vi "Timed Messaging_Skip.vi"(9 "expected":i32=5, 10 "notification":T1=enum."Send next copy now and stop all further copies") -> (3 "Pass?":bool)   [LabVIEW 2014]
uses:
  <vilib>/ActorFramework/Message/Message.lvclass
  <vilib>/ActorFramework/Time-Delayed Send Message/Time-Delay Override Options.ctl
  Increment Msg/Increment Msg.lvclass/Increment Msg.ctl
  <vilib>/ActorFramework/Message Queue/Message Queue.lvclass/Message Queue.ctl
  <vilib>/ActorFramework/Message Dequeuer/Message Dequeuer.lvclass/Message Dequeuer.ctl
  <vilib>/ActorFramework/Message Priority Queue/Priority Dequeue.vi
  Increment Msg/Increment Msg.lvclass
  <vilib>/ActorFramework/Message Queue/Message Queue.lvclass
  <vilib>/ActorFramework/Message Dequeuer/Message Dequeuer.lvclass
panel:
  out "Array":refnum<class "Message.lvclass">[](array[class])
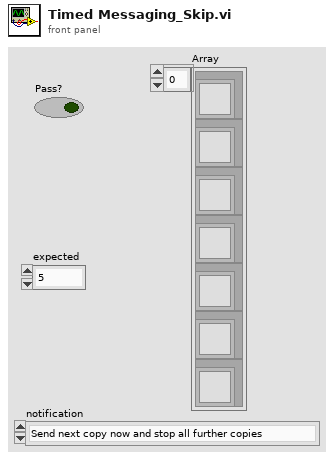
[diagram p1: front panel]
types:
  T1 = typedef "Time-Delay Override Options.ctl" = enum16{"Send next copy now", "Skip next scheduled copy", "Send next copy now and stop all further copies", "Stop all further copies"}
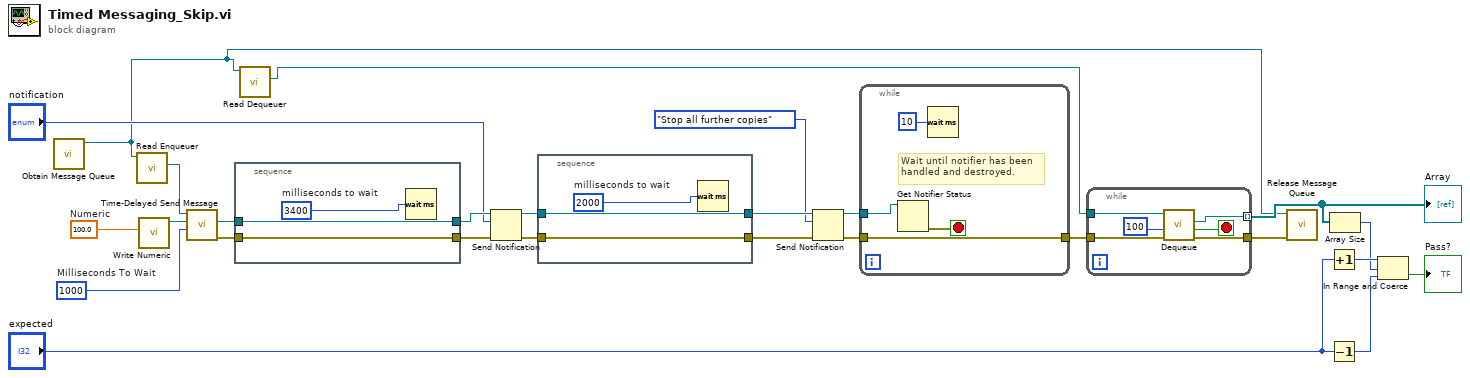
[diagram p0: block diagram]
diagram:
  w24 = 1000  # Milliseconds To Wait
  w26 = 100.0  # Numeric
  n1 = call <vilib>:"Obtain Message Queue.vi"() -> ("Message Queue"=w1:refnum<class "Message Queue.lvclass">)  [unwired: 10 in, 1 out]
  n2 = call <vilib>:"Read Enqueuer.vi"("Message Queue"=w1) -> ("Message Enqueuer"=w4:refnum<class "Message Enqueuer.lvclass">)  [unwired: 10 in]
  n3 = call "Write Numeric.vi"("Numeric"=w26) -> ("Increment Msg out"=w25:refnum<class "Increment Msg.lvclass">)  [unwired: 10 in]
  n4 = call <vilib>:"Time-Delayed Send Message.vi"("Milliseconds To Wait"=w24, "Message"=w25, "Message Enqueuer"=w4) -> ("error out"=w20:errorcluster, "Delivery Notifier"=w23:refnum<notifier>)  [unwired: 7 in]
  n5 = stacked-sequence {
    tunnel: w23 -> [w28]
    tunnel: [w28] -> w22
    tunnel: [w27] -> w21
    tunnel: w20 -> [w27]
    frame #0 {
      w29 = u32 3400  # milliseconds to wait
      n6 = Wait (ms)(milliseconds to wait=w29) -> ()  [unwired: 1 out]
    }
  }
  n7 = call <vilib>:"Read Dequeuer.vi"("Message Queue"=w1) -> ("Message Dequeuer"=w3:refnum<class "Message Dequeuer.lvclass">)  [unwired: 10 in]
  n8 = Send Notification(notification="notification", notifier=w22, error in (no error)=w21) -> (notifier out=w16:refnum<notifier>, error out=w15:errorcluster)
  n9 = stacked-sequence {
    tunnel: w16 -> [w31]
    tunnel: [w31] -> w13
    tunnel: [w30] -> w12
    tunnel: w15 -> [w30]
    frame #0 {
      w32 = u32 2000  # milliseconds to wait
      n10 = Wait (ms)(milliseconds to wait=w32) -> ()  [unwired: 1 out]
    }
  }
  n11 = Send Notification(notification=Time-Delay_Override_Options."Stop all further copies", notifier=w13, error in (no error)=w12) -> (notifier out=w14:refnum<notifier>, error out=w11:errorcluster)
  n12 = while {
    tunnel: w14 -> [w36]
    tunnel: [w34] -> w18
    tunnel: w11 -> [w34]
    stop <- w35 stop-if-true
    # "Wait until notifier has been\nhandled and destroyed."
    n13 = Get Notifier Status(notifier=w36) -> (error out=w35:errorcluster)  [unwired: 1 in, 4 out]
    n14 = Wait (ms)(milliseconds to wait=u32 10) -> ()  [unwired: 1 out]
  }
  n15 = while {
    tunnel: w3 -> [w38]
    tunnel: w18 -> [w42]
    tunnel: [w39] -> w17 mode=indexing
    tunnel: [w41] -> w2
    stop <- w40 stop-if-true
    n16 = call <vilib>:"Dequeue.vi"("error in (no error)"=w42, "timeout in ms (-1)"=100, "Message Dequeuer in"=w38) -> ("error out"=w41:errorcluster, "timed out?"=w40:bool, "Message"=w39:refnum<class "Message.lvclass">)  [unwired: 4 in, 2 out]
  }
  "Array" <- w17
  n17 = call <vilib>:"Release Message Queue.vi"("error in (no error)"=w2, "Message Queue"=w1) -> ()  [unwired: 8 in, 2 out]
  n18 = Increment(x="expected") -> (x+1=w9:i32)
  n19 = Decrement(x="expected") -> (x-1=w8:i32)
  n20 = Array Size(array=w17) -> (size(s)=w6:i32)
  n21 = In Range and Coerce(upper limit=w9, x=w6, lower limit=w8) -> (In Range?=→"Pass?":bool)  [unwired: 1 out]
